vi "Camera Manager Grab Int.vi"(8 "error in (no error)":errorcluster, 9 "imgPtr Input":i32[][](array[numeric]), 11 "cameraId":i32) -> (0 "error out":errorcluster, 2 "imgPtr":i32[][](array[numeric]))   [LabVIEW 2017, in "PlayNitrideCameraComponet1010_4.lvlib"]
doc: "__declspec(dllexport) void CameraManager_Grab_Int(int cameraId, unsigned int* imgPtr);"
uses:
  <userlib>/PlayNitrideCameraComponet1010_4/PlayNitrideCameraComponet1010_4.lvlib
  <userlib>/PlayNitrideCameraComponet1010_4/PlayNitrideCameraComponet.dll
panel:
  out "cameraId 2":i32
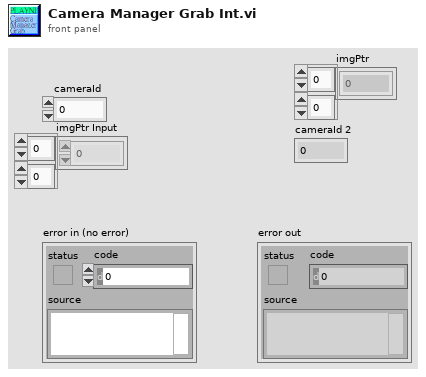
[diagram p1: front panel]
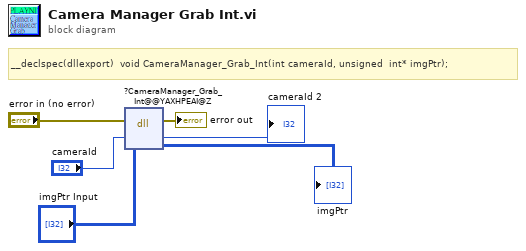
[diagram p0: block diagram]
diagram:
  # "__declspec(dllexport)  void CameraManager_Grab_Int(int cameraId, unsigned  int* imgPtr);"
  n1 = dll-call lib="C:/Program Files/National Instruments/LabVIEW 2017/user.lib/PlayNitrideCameraComponet1010_4/PlayNitrideCameraComponet.*" fn="?CameraManager_Grab_Int@@YAXHPEAI@Z"(error in="error in (no error)", "cameraId"="cameraId", "imgPtr"="imgPtr Input") -> (error out=→"error out":errorcluster, "cameraId"=→"cameraId 2":i32, "imgPtr"=→"imgPtr":u32[][])  [unwired: 3 in, 1 out]
